vi "SAWLAN_EVM_AVG.vi"(8 "error in (no error)":errorcluster, 10 "AvgTimes":i32=1, 11 "VISA resource name":refnum<visa-resource-name>) -> (0 "error out":errorcluster, 3 "VISA resource name out":refnum<visa-resource-name>, 4 "output":T1 {"RMS EVM Avg (dB)" format="%#.3g"; "RMS EVM Avg (%)" format="%#.3g"; "Frequency Error Avg (Hz)" format="%#.3g"; "Avg Burst Power Avg (dBm)" format="%#.3g"})   [LabVIEW 2023, in "Keysight.lvlib"]
uses:
  Keysight.lvlib
panel:
  out "all_data":dbl[](array[numeric])
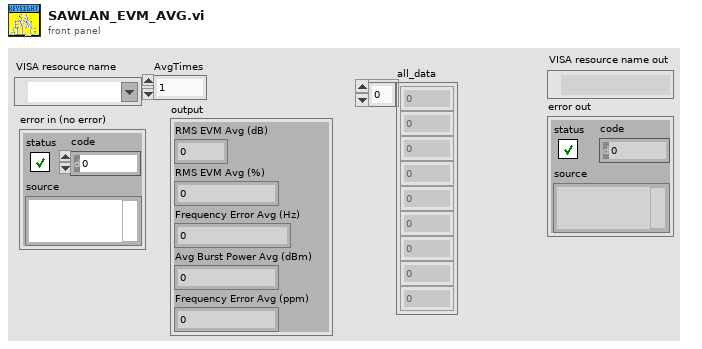
[diagram p1: front panel]
types:
  T1 = cluster{"RMS EVM Avg (dB)":dbl, "RMS EVM Avg (%)":dbl, "Frequency Error Avg (Hz)":dbl, "Avg Burst Power Avg (dBm)":dbl, "Frequency Error Avg (ppm)":dbl}
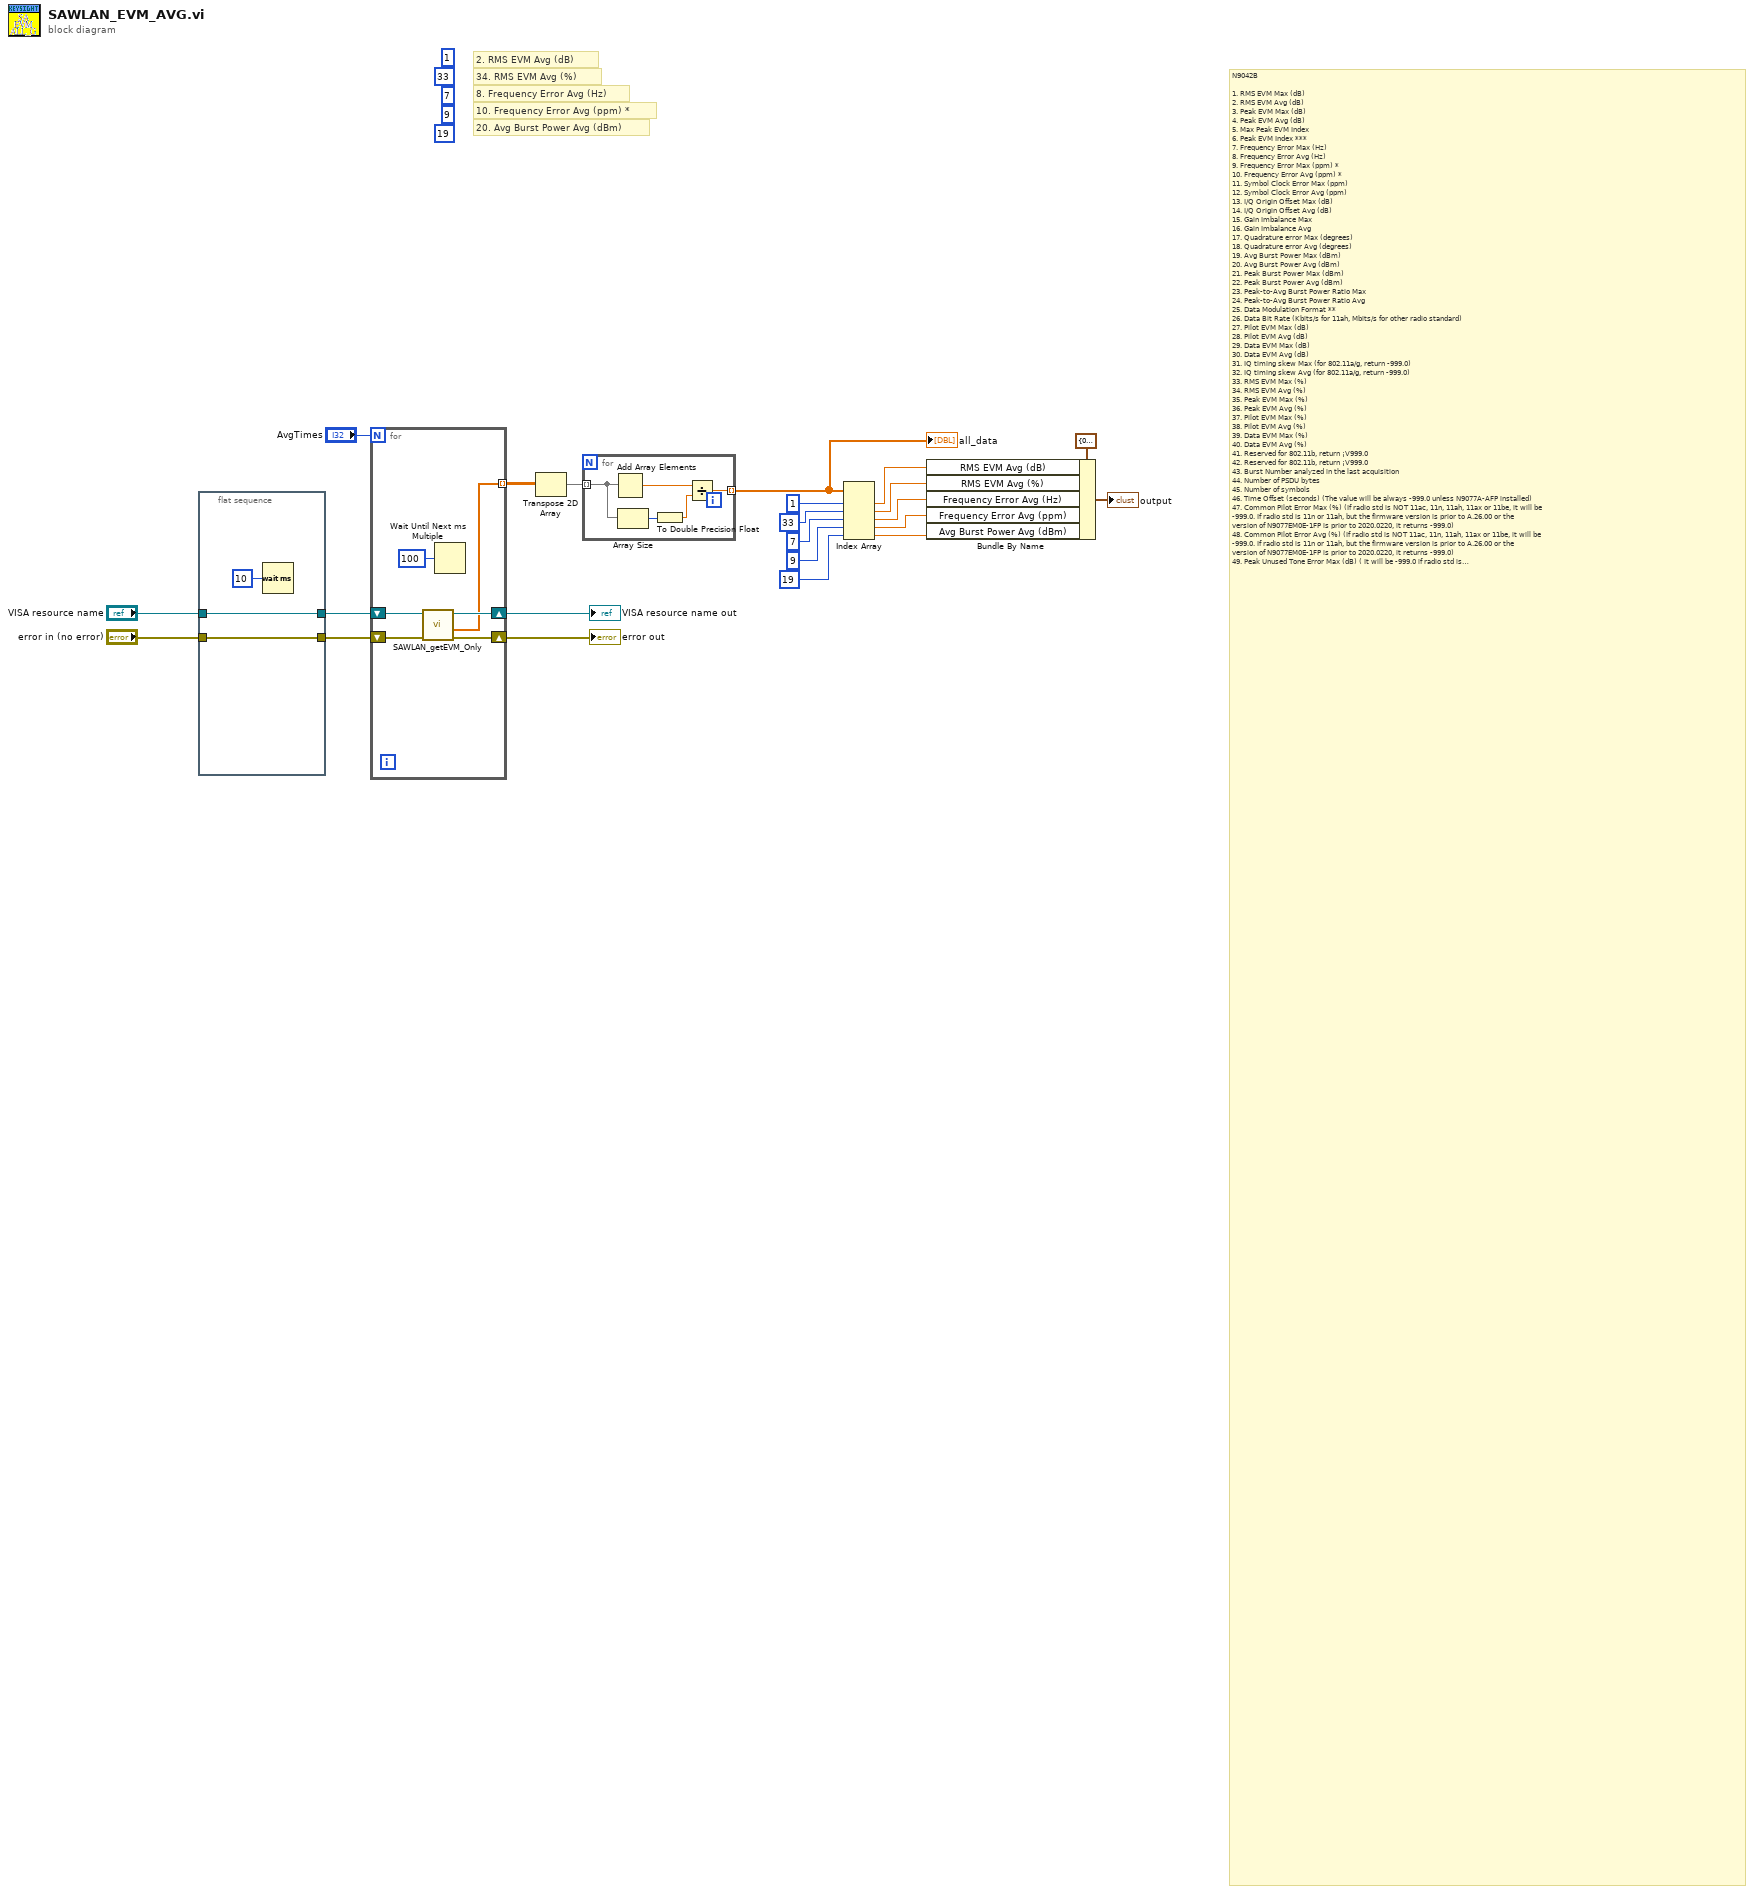
[diagram p0: block diagram]
diagram:
  (unwired) 19 ("index")
  (unwired) 9 ("index")
  (unwired) 7 ("index")
  (unwired) 33 ("index")
  (unwired) 1 ("index")
  # "N9042B\n\n1. RMS EVM Max (dB)\n2. RMS EVM Avg (dB)\n3. Peak EVM Max (dB)\n4. Peak EVM Avg (dB)\n5. Max Peak EVM Index\n6. Peak EVM Index ***\n7. Frequency Error Max (Hz)\n8. Frequency Error Avg (Hz)\n9. Frequency Error Max (ppm) *\n10. Frequency Error Avg (ppm) *\n11. Symbol Clock Error Max (ppm)\n12. Symbol Clock Error Avg (ppm)\n13. I/Q Origin Offset Max (dB)\n14. I/Q Origin Offset Avg (dB)\n15. Gain Imbalance Max\n16. Gain Imbalance Avg\n17. Quadrature error Max (degrees)\n18. Quadrature error Avg (degrees)\n19. Avg Burst Power Max (dBm)\n20. Avg Burst Power Avg (dBm)\n21. Peak Burst Power Max (dBm)\n22. Peak Burst Power Avg (dBm)\n23. Peak-to-Avg Burst Power Ratio Max\n24. Peak-to-Avg Burst Power Ratio Avg\n25. Data Modulation Format **\n26. Data Bit Rate (Kbits/s for 11ah, Mbits/s for other radio standard)\n27. Pilot EVM Max (dB)\n28. Pilot EVM Avg (dB)\n29. Data EVM Max (dB)\n30. Data EVM Avg (dB)\n31. IQ timing skew Max (for 802.11a/g, return -999.0)\n32. IQ timing skew Avg (for 802.11a/g, return -999.0)\n33. RMS EVM Max (%)\n34. RMS EVM Avg (%)\n35. Peak EVM Max (%)\n36. Peak EVM Avg (%)\n37. Pilot EVM Max (%)\n38. Pilot EVM Avg (%)\n39. Data EVM Max (%)\n40. Data EVM Avg (%)\n41. Reserved for 802.11b, return ¡V999.0\n42. Reserved for 802.11b, return ¡V999.0\n43. Burst Number analyzed in the last acquisition\n44. Number of PSDU bytes\n45. Number of symbols\n46. Time Offset (seconds) (The value will be always -999.0 unless N9077A-AFP installed)\n47. Common Pilot Error Max (%) (If radio std is NOT 11ac, 11n, 11ah, 11ax or 11be, it will be\n-999.0. If radio std is 11n or 11ah, but the firmware version is prior to A.26.00 or the\nversion of N9077EM0E-1FP is prior to 2020.0220, it returns -999.0)\n48. Common Pilot Error Avg (%) (If radio std is NOT 11ac, 11n, 11ah, 11ax or 11be, it will be\n-999.0. If radio std is 11n or 11ah, but the firmware version is prior to A.26.00 or the\nversion of N9077EM0E-1FP is prior to 2020.0220, it returns -999.0)\n49. Peak Unused Tone Error Max (dB) ( It will be -999.0 if radio std is NOT 11ax or 11be)\n50. Peak Unused Tone Error Avg (dB) ( It will be -999.0 if radio std is NOT 11ax or 11be)\n51. Symbol Index for Peak Unused Tone Error Max ( It will be -999.0 if radio std is NOT 11ax\nor 11be)\n52. Ru Index for Peak Unused Tone Error Max ( It will be -999.0 if radio std is NOT 11ax or\n11be)\n53. HE/EHT PPDU type ( it is 0~6 and will always be -999 if radio std is NOT 11ax or 11be)\nFor the 53rd result, HE/EHT PPDU type, the returned integer means:\n0 HE_SU\n1 HE_MU\n2 HE_Extended Range SU\n3 HE_TriggerBased\n4 HE_SU_Sounding_NDP\n5 HE_TriggerBased_NDP\n6 EHT_MU\n7 EHT_TriggerBased\n8 EHT_Sounding_NDP\n-999 Unknown\n54. Common Pilot Error Max (Degree) (If radio std is NOT 11ac, 11n, 11ah, 11ax or 11be, it\nwill be -999.0. If radio std is 11n or 11ah, but the firmware version is prior to A.26.00 or\nthe version of N9077EM0E-1FP is prior to 2020.0220, it returns -999.0)\n55. Common Pilot Error Avg (Degree) (If radio std is NOT 11ac, 11n, 11ah, 11ax or 11be, it\nwill be -999.0. If radio std is 11n or 11ah, but the firmware version is prior to A.26.00 or\nthe version of N9077EM0E-1FP is prior to 2020.0220, it returns -999.0)\n56. Packet Extension Duration (us) ( it will be -999.0 if radio std is NOT 11ax or 11be)\n57. Guard Interval of Trigger-based PPDU Guard Interval (us) ( it will be -999.0 if radio std is\nNOT 11ax or 11be)\n58. HE-LTF/EHT-LTF type of Trigger-based PPDU if radio std is 11ax/11be; it will be -999.0\nif radio std is NOT 11ax or 11be\nHE-LTF Type of Trigger-based PPDU, the returned integer means:\n0 1 x LTF\n1 2 x LTF\n2 4 x LTF\nEHT-LTF Type of Trigger-based PPDU, the returned integer means:\n1 2 x LTF\n2 4 x LTF\n59. The minimal Meas Interval for successful PSDU CRC decoding (if the Firmware Version\nis below A.22.00, it returns -999.0 which means Invalid)\n60. PSDU CRC for 802.11a/11n/11ac/11af (if the Firmware Version is below A.22.00 or it is\nnot 802.11a/11n/11ac/11af , 1 means Fail, 0 means Pass, -999 means Invalid)\n61. Duty On Period (Unit is microseconds, it is the pulse width, if the Firmware Version is\nbelow A.30.00 or it is not found, it returns -999.0 which means Invalid.-999.0 means\ninvalid)\n62. Duty Off Period (Unit is microseconds, it is (pulse period ¡V pulse width), if the Firmware\nVersion is below A.30.00 or it is not found, it returns -999.0 which means Invalid.)\n63. Duty Cycle (Unit is %, it is pulse width / pulse period, if the Firmware Version is below\nA.30.00 or (either Duty On or Off is not found), it returns -999.0 which means Invalid\n64. Average RMS ccEVM, if the Firmware Version is below A.33.00 or Cross-Correlated\nEVM is off, it returns -999.0 which means Invalid.\nHere ¡§Average¡¨ means using data of each measurement in measurement loop to\ncalculate RMS ccEVM.\nccEVM is not accurate and can¡¦t reflect source EVM if data point is not sufficient, use\nmore data points (average number * Data Points), then it can lead to a more stable and\naccurate ccEVM result.\nIt will not only benefit for the cases that data point is obviously not sufficient (small BW,\nsmall MCS, small symbol length), for all cases, it will lead to a more accurate ccEVM\nresult, the key point is to balance time and improvement\n65. Valid data points that used to calculate ccEVM, if the Firmware Version is below A.33.00\nor ccEVM is off, it returns -999.0 which means Invalid\n66. Total data points that used to calculate ccEVM, if the Firmware Version is below A.33.00\nor ccEVM is off, it returns -999.0 which means Invalid\n67. Partial Burst Power Max (dBm), if the Firmware Version is below A.36 Minor or Radio Std\nis not 11n/ac/ax/be, returns -999.0, which means Invalid. Valid when Radio Std is 11agjp\nif Radio Std Detection is auto, but invalid if Radio Std Detection is Manual\n68. Partial Burst Power Avg(dBm) if the Firmware Version is below A.36 Minor or Radio Std\nis not 11n/ac/ax/be, returns -999.0, which means Invalid. Valid when Radio Std is 11agjp\nif Radio Std Detection is auto, but invalid if Radio Std Detection is Manual"
  # "34. RMS EVM Avg (%)"
  # "20. Avg Burst Power Avg (dBm)"
  # "10. Frequency Error Avg (ppm) *"
  # "2. RMS EVM Avg (dB)"
  # "8. Frequency Error Avg (Hz)"
  n1 = flat-sequence {
    tunnel: "error in (no error)" -> [w25]
    tunnel: [w25] -> w18
    tunnel: "VISA resource name" -> [w24]
    tunnel: [w24] -> w16
    frame #0 {
      n2 = Wait (ms)(milliseconds to wait=u32 10) -> ()  [unwired: 1 out]
    }
  }
  n3 = for {
    N: "AvgTimes" -> [_]
    shift-right: [w28] -> w22
    shift-left: w16 -> [w29]
    shift-right: [w27] -> w21
    shift-left: w18 -> [w30]
    tunnel: [w26] -> w15 mode=indexing
    n4 = call "SAWLAN_getEVM_Only.vi"("error in"=w30, "VISA in"=w29) -> ("error out"=w27:errorcluster, "All"=w26:dbl[], "VISA out"=w28:refnum<visa-resource-name>)  [unwired: 7 in]
    n5 = Wait Until Next ms Multiple(millisecond multiple=u32 100) -> ()  [unwired: 1 out]
  }
  "VISA resource name out" <- w22
  "error out" <- w21
  n6 = Transpose 2D Array(2D array=w15) -> (transposed array=w14:dbl[][])
  n7 = for {
    tunnel: w14 -> [w33] mode=indexing
    tunnel: [w32] -> w13 mode=indexing
    n8 = Add Array Elements(numeric array=w33) -> (sum=w34:dbl)
    n9 = Array Size(array=w33) -> (size(s)=w35:i32)
    n10 = To Double Precision Float(number=w35) -> (double precision float=w36:dbl)
    n11 = Divide(x=w34, y=w36) -> (x/y=w32:dbl)
  }
  "all_data" <- w13
  n12 = Index Array(array=w13, index #1=1 ("index"), index #2=33 ("index"), index #3=7 ("index"), index #4=9 ("index"), index #5=19 ("index")) -> (element #1=w6:dbl, element #2=w5:dbl, element #3=w4:dbl, element #4=w3:dbl, element #5=w2:dbl)
  n13 = Bundle By Name(cluster=T1 {"RMS EVM Avg (dB)"=0.0, "RMS EVM Avg (%)"=0.0, "Frequency Error Avg (Hz)"=0.0, "Avg Burst Power Avg (dBm)"=0.0, "Frequency Error Avg (ppm)"=0.0} ("get_EVM"), "RMS EVM Avg (dB)"=w6, "RMS EVM Avg (%)"=w5, "Frequency Error Avg (Hz)"=w4, "Frequency Error Avg (ppm)"=w3, "Avg Burst Power Avg (dBm)"=w2) -> (→"output":T1)
